vi "Ball_Teleop.vi"(1 "Joystick_Out":T1) -> ()   [LabVIEW 2018]
uses:
  Utility_VIs/Joystick_Controls.ctl
  Subsytems/Intake_Ball/Intake_Ball_Notifier.ctl
  Subsytems/Intake_Ball/Intake_Ball_Control_Type.ctl
  Global_Variables/Intake_Disc_Globals.vi
  Global_Variables/Intake_Ball_Globals.vi
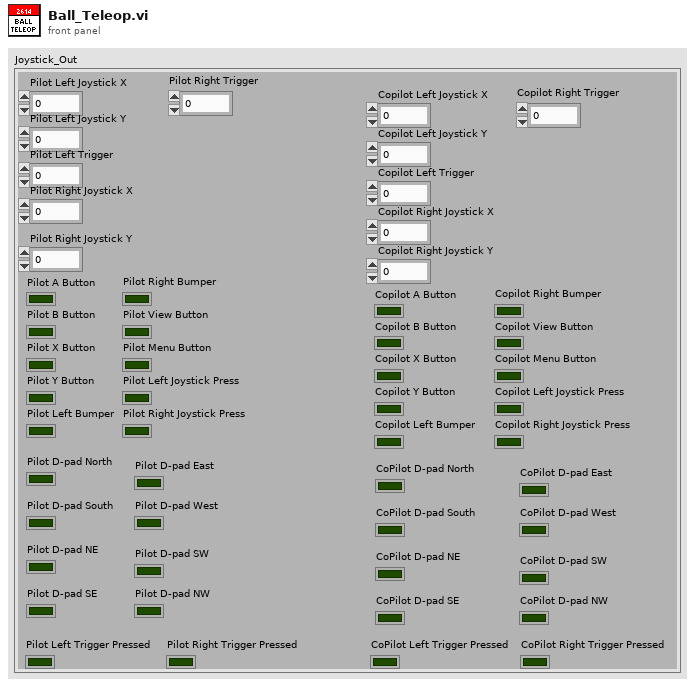
[diagram p1: front panel]
types:
  T1 = typedef "Joystick_Controls.ctl" = cluster{"Pilot Left Joystick X":dbl, "Pilot Left Joystick Y":dbl, "Pilot A Button":bool, "Pilot B Button":bool, "Pilot X Button":bool, "Pilot Y Button":bool, "Pilot Left Bumper":bool, "Pilot Right Bumper":bool, "Pilot View Button":bool, "Pilot Menu Button":bool, "Pilot Left Joystick Press":bool, "Pilot Right Joystick Press":bool, "Pilot Left Trigger":dbl, "Pilot Right Joystick X":dbl, "Pilot Right Joystick Y":dbl, "Pilot Right Trigger":dbl, "Copilot Left Joystick X":dbl, "Copilot Left Joystick Y":dbl, "Copilot A Button":bool, "Copilot B Button":bool, "Copilot X Button":bool, "Copilot Y Button":bool, "Copilot Left Bumper":bool, "Copilot Right Bumper":bool, "Copilot View Button":bool, "Copilot Menu Button":bool, "Copilot Left Joystick Press":bool, "Copilot Right Joystick Press":bool, "Copilot Left Trigger":dbl, "Copilot Right Joystick X":dbl, "Copilot Right Joystick Y":dbl, "Copilot Right Trigger":dbl, "Pilot D-pad North":bool, "Pilot D-pad South":bool, "Pilot D-pad East":bool, "Pilot D-pad West":bool, "Pilot D-pad NE ":bool, "Pilot D-pad SE":bool, "Pilot D-pad SW":bool, "Pilot D-pad NW":bool, "CoPilot D-pad North":bool, "CoPilot D-pad South":bool, "CoPilot D-pad East":bool, "CoPilot D-pad West":bool, "CoPilot D-pad NE":bool, "CoPilot D-pad SE":bool, "CoPilot D-pad SW":bool, "CoPilot D-pad NW":bool, "Pilot Left Trigger Pressed":bool, "Pilot Right Trigger Pressed":bool, "CoPilot Left Trigger Pressed":bool, "CoPilot Right Trigger Pressed":bool}
  T2 = typedef "Intake_Ball_Notifier.ctl" = cluster{"Intake_Ball_Control_Type":T3, "Manual_In":bool, "Manual_Out":bool, "Ball_In":bool, "Ball_Out":bool, "Parameter_One":dbl, "Parameter_Two":dbl, "Parameter_Three":dbl, "Step":i32, "Ball_Notifier":refnum<notifier>}
  T3 = typedef "Intake_Ball_Control_Type.ctl" = enum16{"No_Op", "Manual_In", "Manual_Out", "In_Sensor_Stop", "Out_Teleop", "Out", "Stall"}
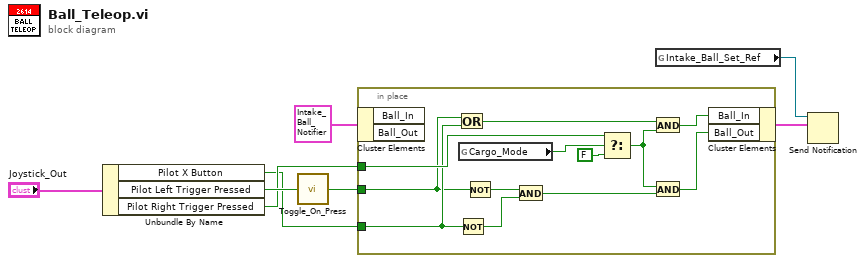
[diagram p0: block diagram]
diagram:
  n1 = Unbundle By Name("Joystick_Out") -> ("Pilot X Button"=w1:bool, "Pilot Left Trigger Pressed"=w5:bool, "Pilot Right Trigger Pressed"=w4:bool)
  n2 = call "Toggle_On_Press.vi"("Boolean"=w5) -> ("Boolean Out"=w2:bool)
  n3 = in-place {
    in-place-border: w4 -> [w16]
    in-place-border: w2 -> [w10]
    in-place-border: w1 -> [w12]
    n4 = in-place-cluster #1(T2 {"Intake_Ball_Control_Type"=enum."No_Op", "Manual_In"=FALSE, "Manual_Out"=FALSE, "Ball_In"=FALSE, "Ball_Out"=FALSE, "Parameter_One"=0.0, "Parameter_Two"=0.0, "Parameter_Three"=0.0, "Step"=0, "Ball_Notifier"=refnum} ("Intake_Ball_Notifier")) -> ()  [unwired: 2 out]
    n5 = Or(x=w10, y=w12) -> (x .or. y?=w13:bool)
    n6 = Not(x=w12) -> (.not. x?=w11:bool)
    n7 = global read "Intake_Disc_Globals.vi" "Cargo_Mode"() -> (w20:bool)
    n8 = Not(x=w10) -> (.not. x?=w9:bool)
    n9 = And(x=w9, y=w11) -> (x .and. y?=w14:bool)
    n10 = Select(t=w16, s=w20, f=FALSE) -> (s? t:f=w17:bool)
    n11 = And(x=w13, y=w17) -> (x .and. y?=w18:bool)
    n12 = And(x=w17, y=w14) -> (x .and. y?=w19:bool)
    n13 = in-place-cluster #1("Ball_In"=w18, "Ball_Out"=w19) -> (w8:T2)
  }
  n14 = global read "Intake_Ball_Globals.vi" "Intake_Ball_Set_Ref"() -> (w3:refnum<notifier>)
  n15 = Send Notification(notification=w8, notifier=w3) -> ()  [unwired: 1 in, 2 out]
